vi "Send Add Event.vi"(7 "Priority":T1=enum."Normal" caption="Message Priority (Normal)", 8 "error in (no error)":errorcluster, 9 "Controller Event Handler":refnum<class "Abstract Event Handler for Controller.lvclass">, 10 "Event":refnum<class "Event.lvclass">, 11 "Message Enqueuer in":refnum<class "Message Enqueuer.lvclass">) -> (0 "error out":errorcluster, 3 "Message Enqueuer out":refnum<class "Message Enqueuer.lvclass">)   [LabVIEW 2023, in "MVC Actors.lvlib" / "Add Event Msg.lvclass"]
doc: "Sends the <b>MVC Actors.lvlib:Add Event Msg.lvclass</b> message.\n\nThis message will call <b>Add Event.vi</b> on the <b>MVC Actors.lvlib:Controller.lvclass</b> actor.\n\n<b>Add Event.vi Description</b>\nThis method adds an event to the list of the events handled by the Controller Actor. If the Controller Actor wants to handle the events from the View, a concrete implementation of the <b>\"Abstract Event Handler for Controller.lvclass\"</b> should be wired to the <b>\"Controller Event Handler\"</b> terminal."
uses:
  Add Event Msg.lvclass
  Add Event Msg.lvclass/Add Event Msg.ctl
  <vilib>/ActorFramework/Message Enqueuer/Message Enqueuer.lvclass
  C:/Program Files/National Instruments/LabVIEW 2023/vi.lib/ActorFramework/Message/Message.lvclass
  C:/Projects/Shared Libraries/Event Actors/Controller Messages/Add Event Msg/Add Event Msg.lvclass
  <vilib>/ActorFramework/Message Enqueuer/Message Priority.ctl
  Event/Event.lvclass
  Event Handlers/Abstract Event Handler for Controller/Abstract Event Handler for Controller.lvclass
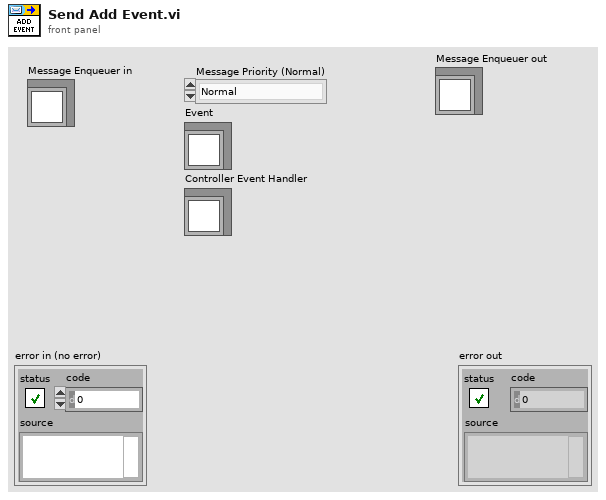
[diagram p1: front panel]
types:
  T1 = typedef "Actor Framework.lvlib/Message Enqueuer.lvclass/Message Priority.ctl" = enum16{"Low", "Normal", "High"}
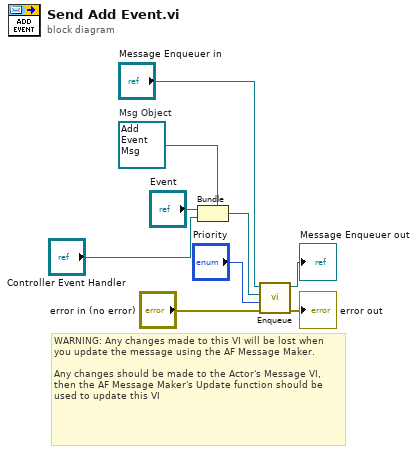
[diagram p0: block diagram]
diagram:
  w7 = refnum<class "Add Event Msg.lvclass"> refnum  # Msg Object
  # "WARNING: Any changes made to this VI will be lost when you update the message using the AF Message Maker.\n\nAny changes should be made to the Actor's Message VI, then the AF Message Maker's Update function should be used to update this VI"
  n1 = Bundle(cluster=w7, "Event", "Controller Event Handler") -> (w2:refnum<class "Add Event Msg.lvclass">)
  n2 = call <vilib>:"Enqueue.vi"("error in (no error)"="error in (no error)", "Message Priority (Normal)"="Priority", "Message"=w2, "Message Enqueuer in"="Message Enqueuer in") -> ("error out"=→"error out":errorcluster, "Message Enqueuer out"=→"Message Enqueuer out":refnum<class "Message Enqueuer.lvclass">)  [unwired: 6 in]
